vi "gentec-M-Link.Test.vi"(0 "VISA resource In":refnum<visa-resource-name>, 2 "Data to Write":string="N/A", 5 "error in (no error)":errorcluster) -> (13 "Read Timeout":bool, 14 "VISA resource Out":refnum<visa-resource-name>, 15 "Data Read":string, 19 "error out":errorcluster)   [LabVIEW 2014, in "gentec-M-Link - Driver.lvlib"]
doc: "This is a simple test VI: It sends \"Data to write\" by a VISA write command to the device, waits a certain time, and reads the data published by the device."
uses:
  gentec-M-Link - Driver.lvlib
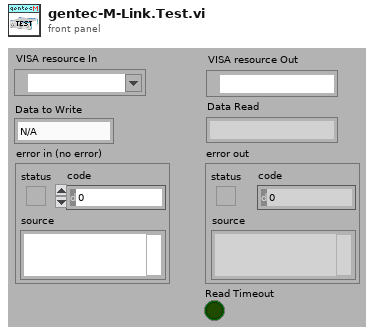
[diagram p1: front panel]
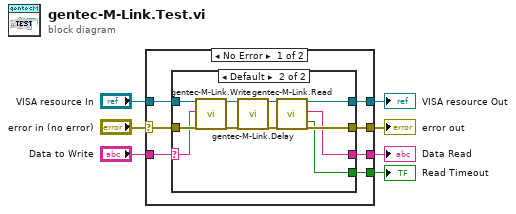
[diagram p0: block diagram]
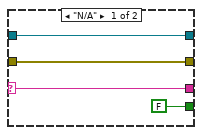
[diagram p2: hidden frame]
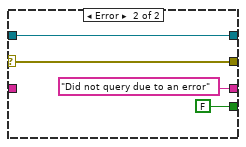
[diagram p3: hidden frame]
diagram:
  n1 = case shown="No Error" "error in (no error)" {
    selector: "error in (no error)" -> [w13 w33]
    tunnel: [w14 w33] -> w6
    tunnel: "VISA resource In" -> [w12 w32]
    tunnel: [w11 w32] -> w4
    tunnel: [w10 "Did not query due to an error" ("Data Read")] -> w3
    tunnel: [w9 FALSE ("Read Timeout")] -> w2
    tunnel: "Data to Write" -> [w8 _]
    frame No Error {
      n2 = case shown="Default" w8 {
        selector: w8 -> [w17 w19]
        tunnel: [w16 w29] -> w14
        tunnel: w13 -> [w16 w28]
        tunnel: w12 -> [w18 w27]
        tunnel: [w18 w25] -> w11
        tunnel: [w17 w24] -> w10
        tunnel: [FALSE ("Read Timeout") w23] -> w9
        frame "N/A" {
        }
        frame Default {
          n3 = call "gentec-M-Link.Write.vi"("VISA resource (In)"=w27, "Data To Write"=w19, "error in (no error)"=w28) -> ("VISA resource (Out)"=w21:refnum<visa-resource-name>, "error out"=w26:errorcluster)  [unwired: 14 in, 1 out]
          n4 = call "gentec-M-Link.Delay.vi"("VISA resource In"=w21, "error in (no error)"=w26) -> ("VISA resource Out"=w20:refnum<visa-resource-name>, "error out"=w22:errorcluster)  [unwired: 16 in]
          n5 = call "gentec-M-Link.Read.vi"("VISA resource (In)"=w20, "error in (no error)"=w22) -> ("VISA resource (Out)"=w25:refnum<visa-resource-name>, "Data Read"=w24:string, "Read Timeout"=w23:bool, "error out"=w29:errorcluster)  [unwired: 13 in, 1 out]
        }
      }
    }
    frame Error {
    }
  }
  "error out" <- w6
  "VISA resource Out" <- w4
  "Data Read" <- w3
  "Read Timeout" <- w2
